vi "MainXRF.vi"() -> ()   [LabVIEW 2023]
panel:
  in  "path folder tabs":path
  in  "Type Tables":enum32{"Item 0", "Item 1"}(radio)
  in  "figs":bool
  in  "mapping":bool
  in  "xrf":bool
  in  "Stop":bool
  out "error out":errorcluster
  in  "error in":errorcluster
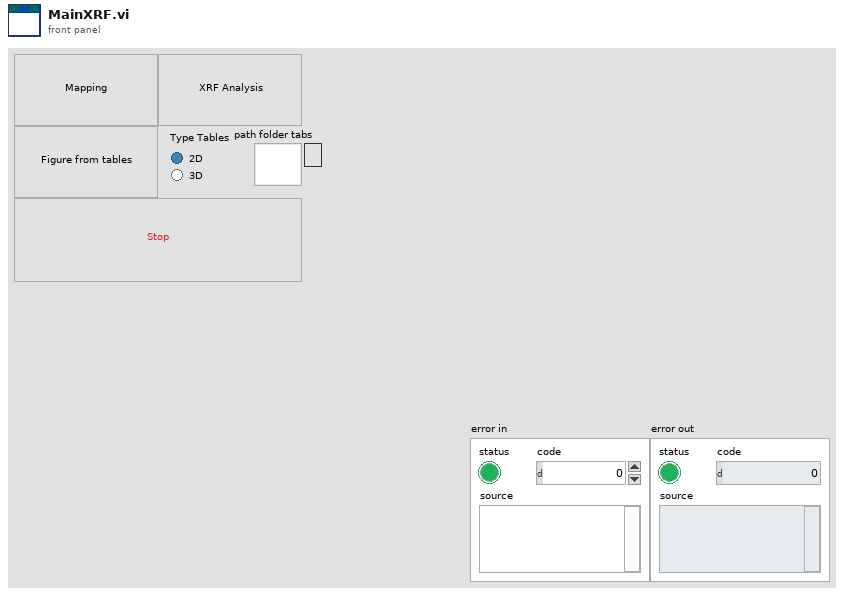
[diagram p1: front panel]
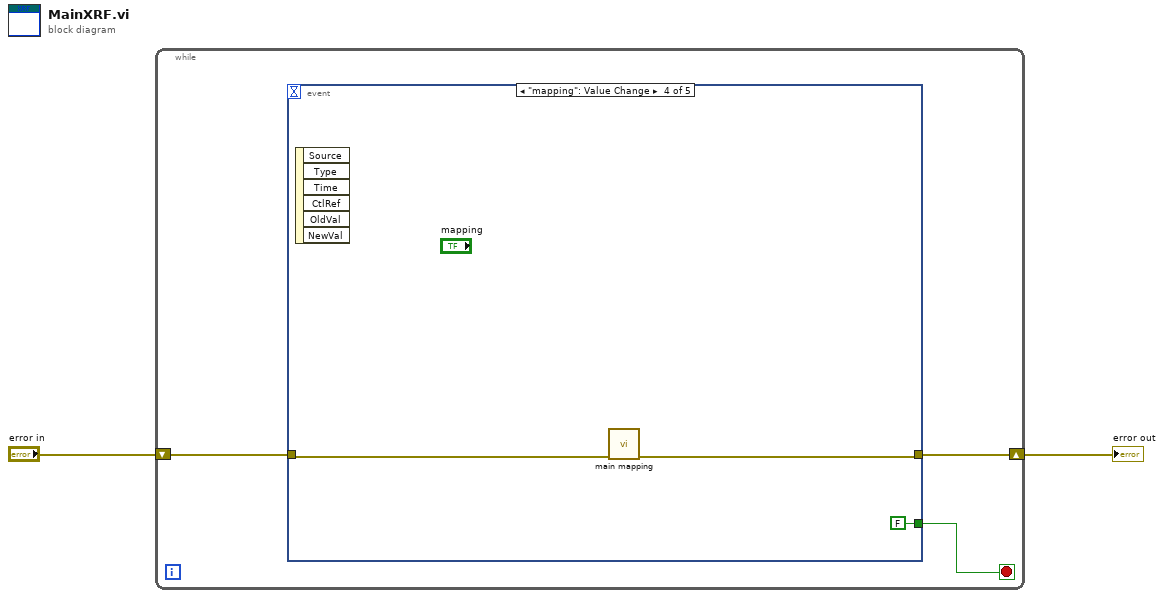
[diagram p0: block diagram]
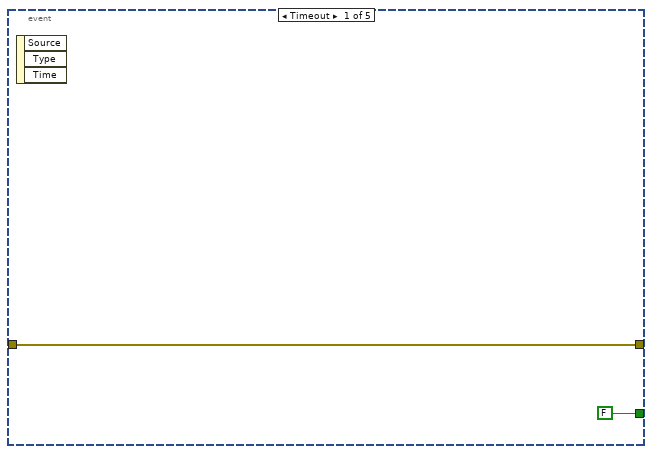
[diagram p2: hidden frame]
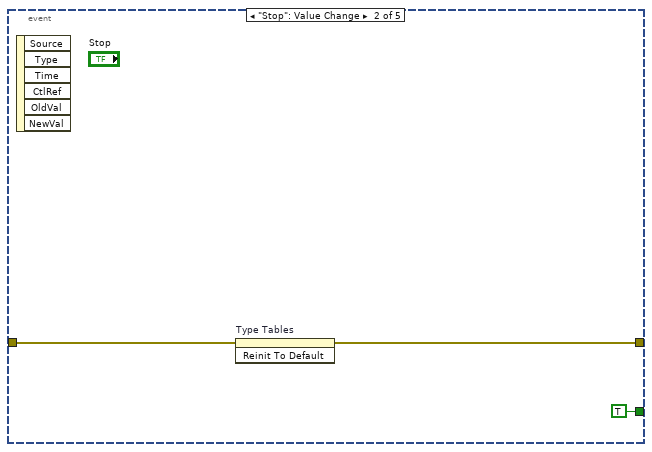
[diagram p3: hidden frame]
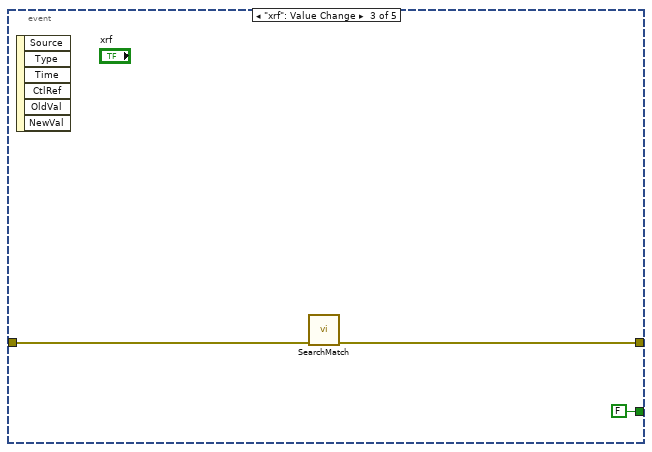
[diagram p4: hidden frame]
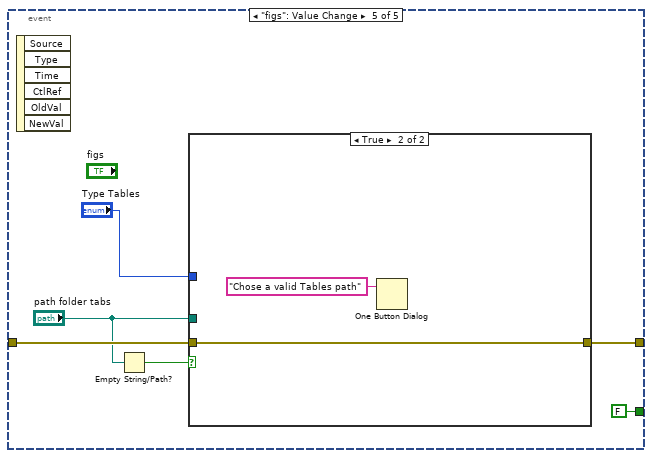
[diagram p5: hidden frame]
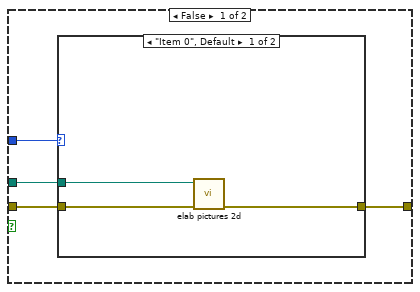
[diagram p6: hidden frame]
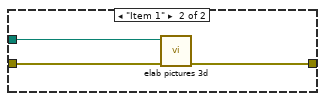
[diagram p7: hidden frame]
diagram:
  n1 = while {
    shift-right: [w3] -> w1
    shift-left: "error in" -> [w4]
    stop <- w5 stop-if-true
    n2 = event shown="[3] \"mapping\": Value Change" {
      selector: _ -> [_ _ _ _ _]
      dyn-events: _ -> [_ _ _ _ _]
      timeout: _ -> [_ _ _ _ _]
      tunnel: [FALSE TRUE FALSE FALSE FALSE] -> w5
      tunnel: w4 -> [w6 w9 w13 w15 w21]
      tunnel: [w6 w8 w12 w14 w20] -> w3
      event Timeout {
        n3 = event-data() -> ()  [unwired: 1 in, 3 out]
      }
      event "Stop": Value Change {
        n4 = event-data() -> ()  [unwired: 1 in, 6 out]
        n5 = invoke on="Type Tables" class="RadioBtnsControl (strict)" method="Reinit To Default"(error in=w9) -> (error out=w8:errorcluster)  [unwired: 2 in, 2 out]
      }
      event "xrf": Value Change {
        n6 = event-data() -> ()  [unwired: 1 in, 6 out]
        n7 = call "SearchMatch.vi"("Error In"=w13) -> ("Error Out"=w12:errorcluster)  [unwired: 6 in, 4 out]
      }
      event "mapping": Value Change {
        n8 = event-data() -> ()  [unwired: 1 in, 6 out]
        n9 = call "main mapping.vi"("error in"=w15) -> ("error out"=w14:errorcluster)  [unwired: 10 in]
      }
      event "figs": Value Change {
        n10 = event-data() -> ()  [unwired: 1 in, 6 out]
        n11 = Empty String/Path?(string/path="path folder tabs") -> (empty?=w18:bool)
        n12 = case shown="True" w18 {
          tunnel: "Type Tables" -> [w26 _]
          tunnel: w21 -> [w25 w34]
          tunnel: [w24 w34] -> w20
          tunnel: "path folder tabs" -> [w23 _]
          frame False {
            n13 = case shown="\"Item 0\", Default" w26 {
              tunnel: w25 -> [w29 w32]
              tunnel: [w28 w31] -> w24
              tunnel: w23 -> [w27 w30]
              frame "Item 0", Default {
                n14 = call "elab pictures 2d.vi"("error in"=w29, "path file in"=w27) -> ("error out"=w28:errorcluster)  [unwired: 9 in]
              }
              frame "Item 1" {
                n15 = call "elab pictures 3d.vi"("error in"=w32, "path file in"=w30) -> ("error out"=w31:errorcluster)  [unwired: 9 in]
              }
            }
          }
          frame True {
            n16 = One Button Dialog(message="Chose a valid Tables path") -> ()  [unwired: 1 in, 1 out]
          }
        }
      }
    }
  }
  "error out" <- w1
